vi "GetControlRefByName.vi"(7 "VI输入":refnum<vi>, 10 "错误输入（无错误）":errorcluster, 11 "控件名":string) -> (2 "错误输出":errorcluster, 3 "控件输出":refnum<vi>)   [LabVIEW 2020]
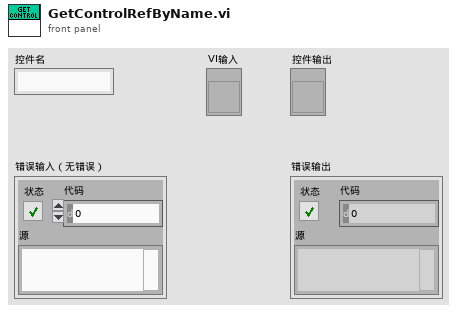
[diagram p1: front panel]
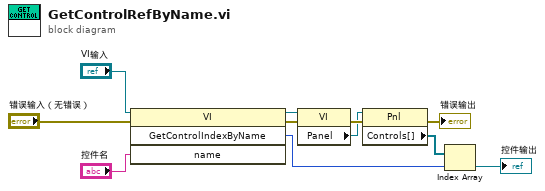
[diagram p0: block diagram]
diagram:
  n1 = invoke class="VI" method="GetControlIndexByName"(reference="VI输入", error in="错误输入（无错误）", "name"="控件名") -> (reference out=w3:refnum<vi>, error out=w8:errorcluster, "GetControlIndexByName"=w6:i32)  [unwired: 1 in, 1 out]
  n2 = property class="VI"(reference=w3, error in=w8) -> (error out=w9:errorcluster, "Panel"=w4:refnum<vi>)  [unwired: 1 out]
  n3 = property class="Pnl"(reference=w4, error in=w9) -> (error out=→"错误输出":errorcluster, "Controls[]"=w5:refnum<vi>[])  [unwired: 1 out]
  n4 = Index Array(array=w5, index=w6) -> (element=→"控件输出":refnum<vi>)
